vi "探头窗口-24-4列.vi"() -> ()   [LabVIEW 2017]
panel:
  in  "更新数据":T1
  in  "停止信号":bool=TRUE
  out "更新数据？":bool=TRUE
  out "引用-切回列表模式？":refnum<vi>
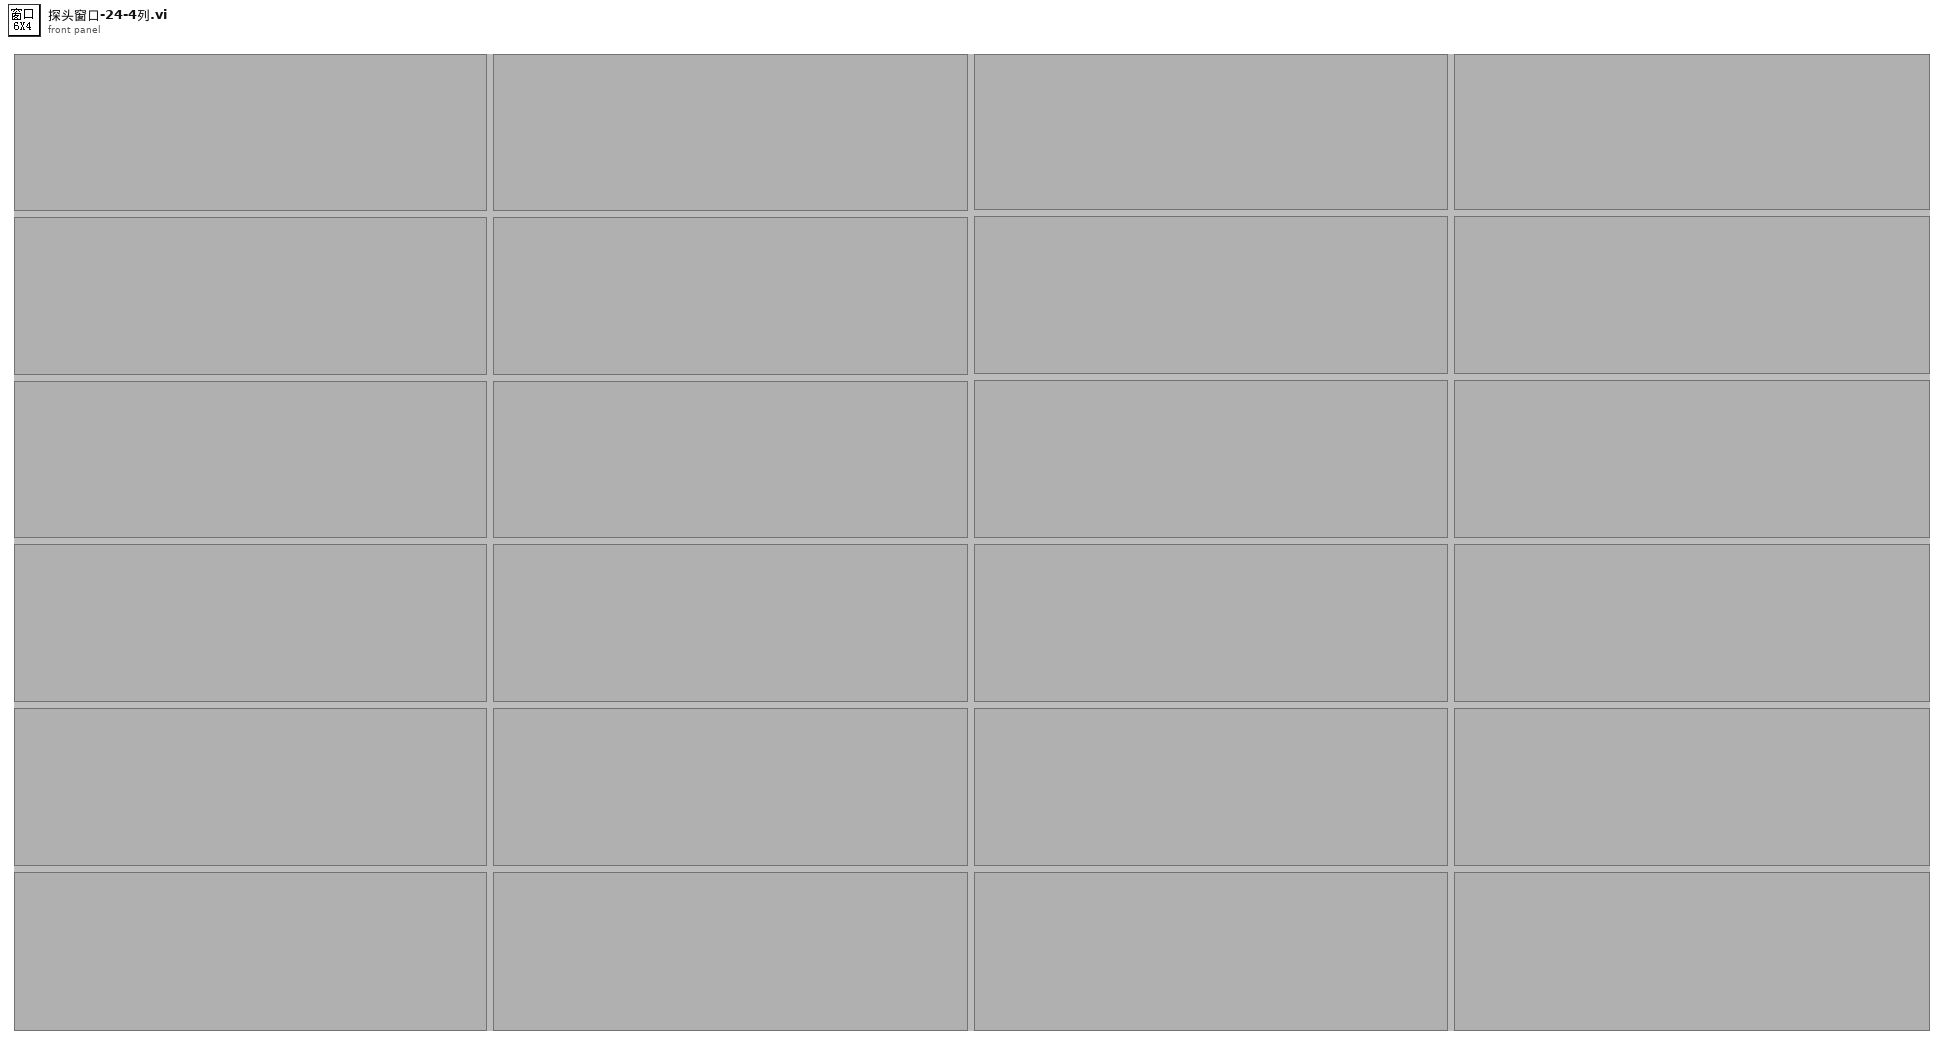
[diagram p1: front panel]
types:
  T1 = cluster{"探头启用状态？":bool[], "测量值":cluster{"X":timestamp, "Y":dbl}[], "限值":cluster{"限值1":dbl, "限值2":dbl, "探头限值":enum16{"一级限值", "二级限值"}}[], "报警状态":enum16{"正常", "一级报警", "二级报警", "累积报警"}[], "探头信息":string[], "累积剂量":cluster{"设备名称":string, "启用累积？":bool, "起始时间":timestamp, "累积剂量":dbl, "累积报警阈值":dbl}[]}
  T2 = cluster{"启用状态？":bool, "测量值":cluster{"X":timestamp, "Y":dbl}, "限值簇":cluster{"限值1":dbl, "限值2":dbl, "探头限值":enum16{"一级限值", "二级限值"}}, "报警状态":enum16{"正常", "一级报警", "二级报警", "累积报警"}, "探头信息":string, "探头地址":i32, "累积剂量":cluster{"设备名称":string, "启用累积？":bool, "起始时间":timestamp, "累积剂量":dbl, "累积报警阈值":dbl}}
  T3 = typedef "eventvkey.ctl" = enum16{"ASCII", "Enter", "Return", "Shift", "Ctrl", "Alt", "Cmd", "Opt", "Caps", "NumLock", "Clear", "Break", "Up", "Down", "Left", "Right", "Insert", "Delete", "Home", "End", "PageUp", "PageDown", "Escape", "Help", "Pause", "ScrollLock", "F1", "F2", "F3", "F4", "F5", "F6", "F7", "F8", "F9", "F10", "F11", "F12", "F13", "F14", "F15", "F16", "F17", "F18", "F19", "F20", "F21", "F22", "F23", "F24", "Play", "VolumeUp", "VolumeDown", "Mute", "Two Byte Char"}
  T4 = cluster{"限值1":dbl, "限值2":dbl, "探头限值":enum16{"一级限值", "二级限值"}}
  T5 = cluster{"限值1":dbl, "限值2":dbl, "探头限值":enum16{"一级限值", "二级限值"}}[]
  T6 = cluster{"设备名称":string, "启用累积？":bool, "起始时间":timestamp, "累积剂量":dbl, "累积报警阈值":dbl}[]
  T7 = cluster{"设备名称":string, "启用累积？":bool, "起始时间":timestamp, "累积剂量":dbl, "累积报警阈值":dbl}
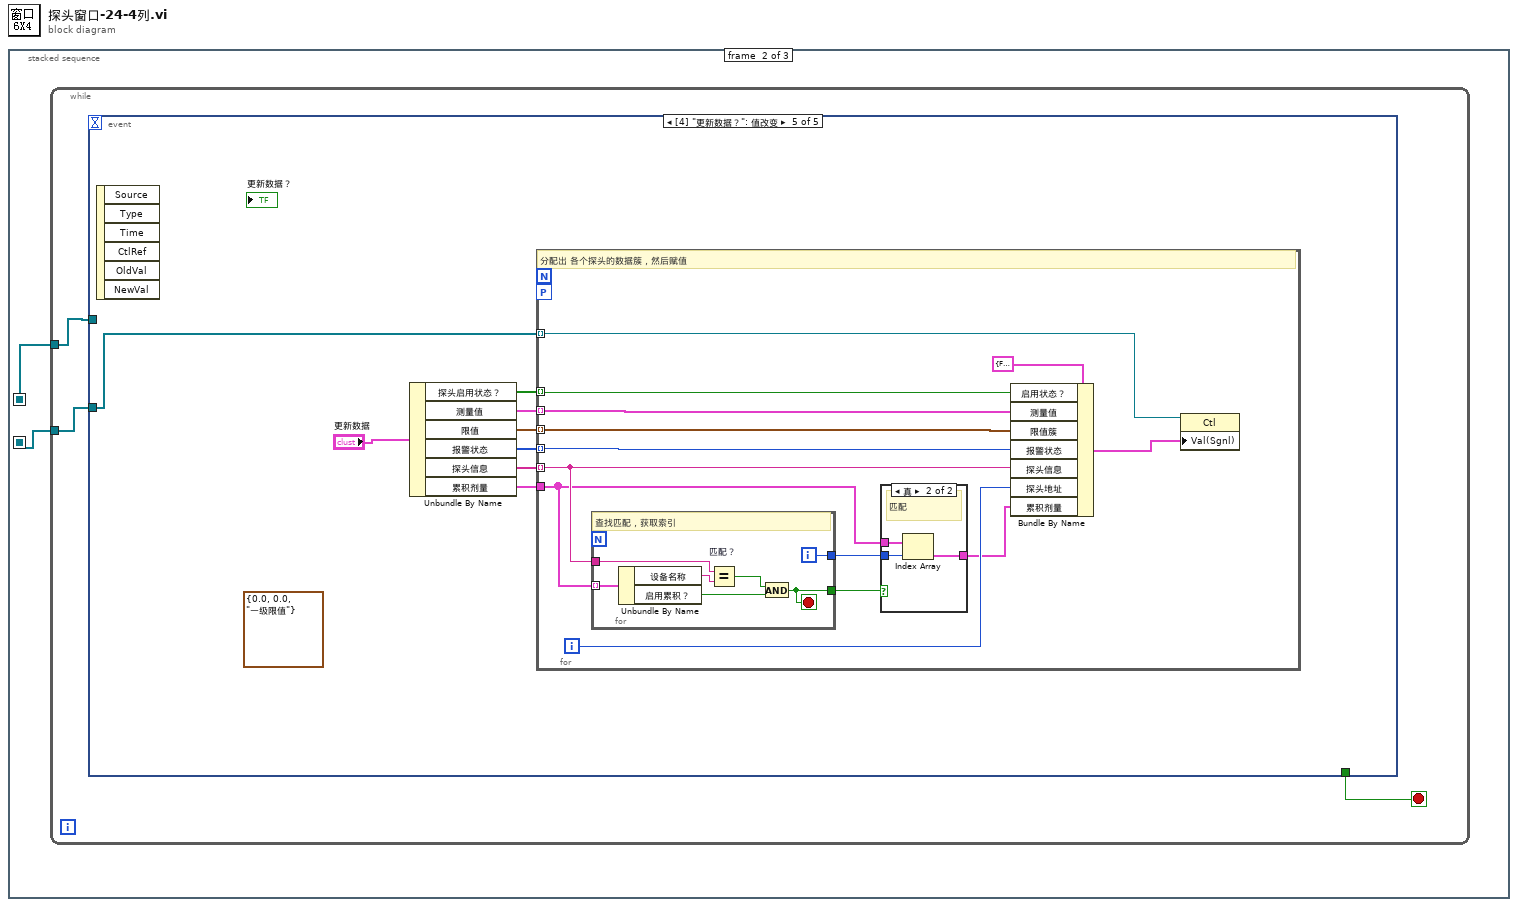
[diagram p0: block diagram]
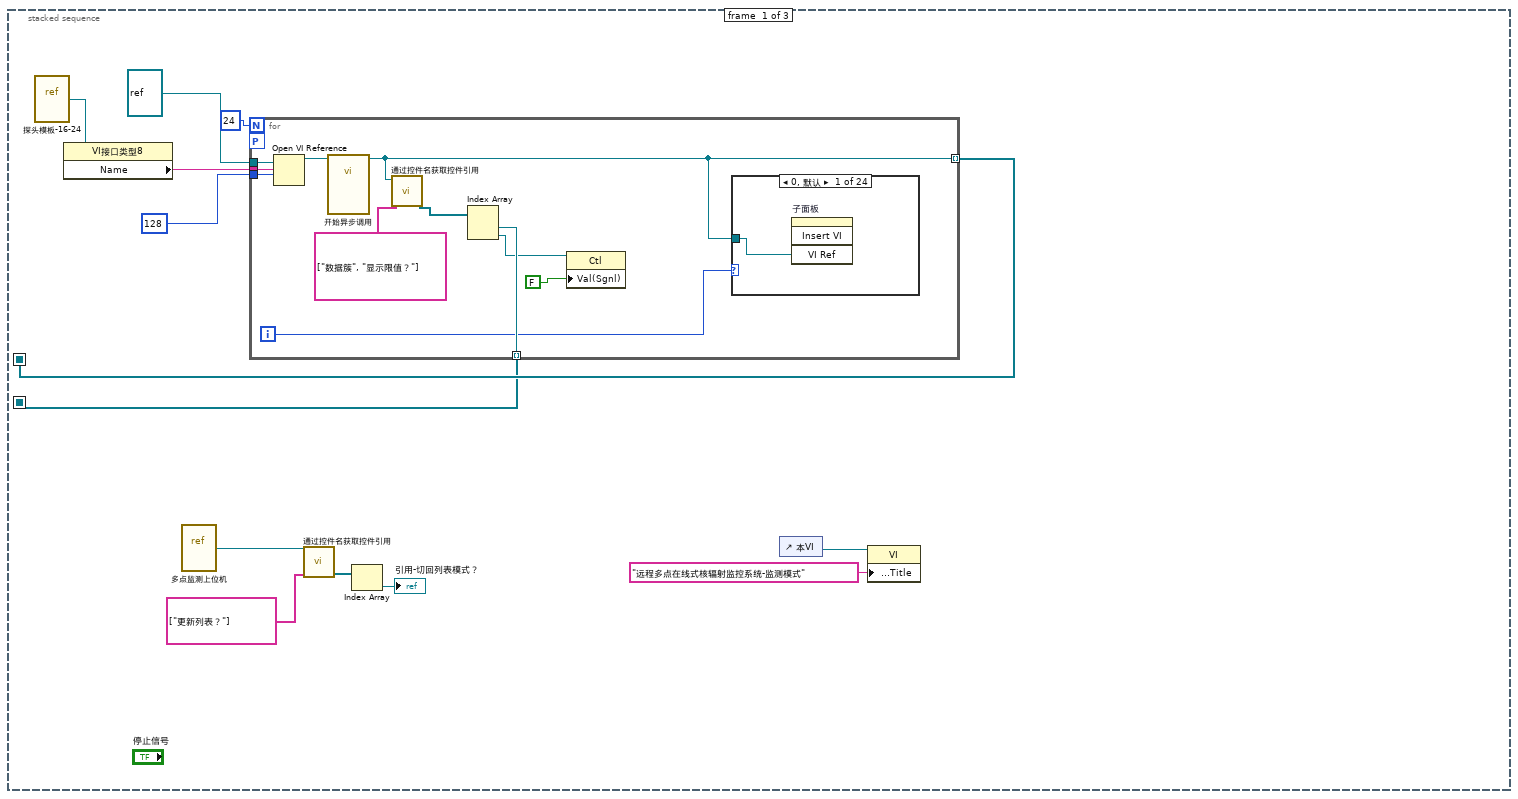
[diagram p2: hidden frame]
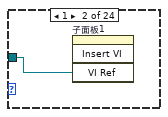
[diagram p3: hidden frame]
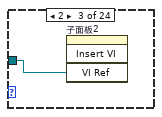
[diagram p4: hidden frame]
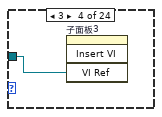
[diagram p5: hidden frame]
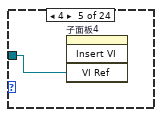
[diagram p6: hidden frame]
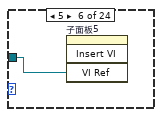
[diagram p7: hidden frame]
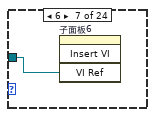
[diagram p8: hidden frame]
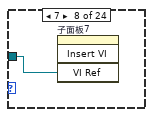
[diagram p9: hidden frame]
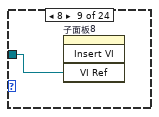
[diagram p10: hidden frame]
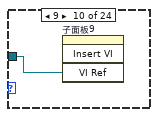
[diagram p11: hidden frame]
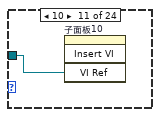
[diagram p12: hidden frame]
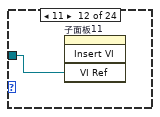
[diagram p13: hidden frame]
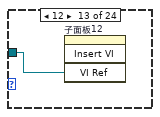
[diagram p14: hidden frame]
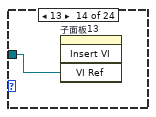
[diagram p15: hidden frame]
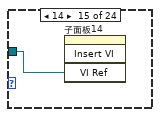
[diagram p16: hidden frame]
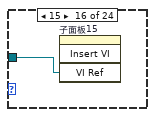
[diagram p17: hidden frame]
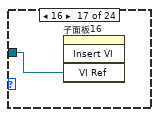
[diagram p18: hidden frame]
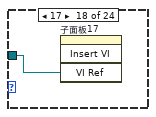
[diagram p19: hidden frame]
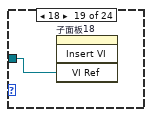
[diagram p20: hidden frame]
diagram:
  n1 = stacked-sequence {
    seq-local: [w8 _ _] -> [_ w50 _]
    seq-local: [w7 _ _] -> [_ w49 _]
    frame #0 {
      n2 = vi-ref "探头模板-16-24.vi"() -> (w13:refnum<vi>)
      n3 = property class="VI接口类型8"(reference=w13) -> ("Name"=w12:string)  [unwired: 1 in, 2 out]
      n4 = vi-ref "多点监测上位机.vi"() -> (w3:refnum<vi>)
      n5 = for {
        N: 24 -> [_]
        tunnel: w12 -> [w24]
        tunnel: 128 ("选项") -> [w23]
        tunnel: refnum<vi> refnum ("类型说明符VI引用句柄（仅用于类型）") -> [w22]
        tunnel: [w16] -> w8 mode=indexing
        tunnel: [w19] -> w7 mode=indexing
        workers-P: _ -> [_]
        i -> [w18]
        n6 = Open VI Reference(type specifier VI Refnum (for type only)=w22, vi path=w24, options=w23) -> (vi reference=w17:refnum<vi>)  [unwired: 3 in, 1 out]
        n7 = call-by-ref "开始异步调用"(reference=w17) -> (reference out=w16:refnum<vi>)  [unwired: 13 in, 1 out]
        n8 = call "通过控件名获取控件引用.vi"("控件名数组"=string[] ["数据簇", "显示限值？"], "VI引用"=w16) -> ("控件引用输出"=w21:refnum<vi>[])  [unwired: 7 in, 2 out]
        n9 = Index Array(array=w21) -> (element #1=w19:refnum<vi>, element #2=w15:refnum<vi>)  [unwired: 2 in]
        n10 = property class="Ctl"(reference=w15, "Val(Sgnl)"=FALSE ("显示报警限值？")) -> ()  [unwired: 1 in, 2 out]
        n11 = case shown="0, 默认" w18 {
          tunnel: w16 -> [w25 w26 w27 w28 w29 w30 w31 w32 w33 w34 w35 w36 w37 w38 w39 w40 w41 w42 w43 w44 w45 w46 w47 w48]
          frame 0, Default {
            n12 = invoke on="子面板" class="子面板" method="Insert VI"("VI Ref"=w25) -> ()  [unwired: 3 in, 4 out]
          }
          frame 1 {
            n13 = invoke on="子面板1" class="SubPnl" method="Insert VI"("VI Ref"=w26) -> ()  [unwired: 3 in, 4 out]
          }
          frame 2 {
            n14 = invoke on="子面板2" class="SubPnl" method="Insert VI"("VI Ref"=w27) -> ()  [unwired: 3 in, 4 out]
          }
          frame 3 {
            n15 = invoke on="子面板3" class="SubPnl" method="Insert VI"("VI Ref"=w28) -> ()  [unwired: 3 in, 4 out]
          }
          frame 4 {
            n16 = invoke on="子面板4" class="SubPnl" method="Insert VI"("VI Ref"=w29) -> ()  [unwired: 3 in, 4 out]
          }
          frame 5 {
            n17 = invoke on="子面板5" class="SubPnl" method="Insert VI"("VI Ref"=w30) -> ()  [unwired: 3 in, 4 out]
          }
          frame 6 {
            n18 = invoke on="子面板6" class="SubPnl" method="Insert VI"("VI Ref"=w31) -> ()  [unwired: 3 in, 4 out]
          }
          frame 7 {
            n19 = invoke on="子面板7" class="SubPnl" method="Insert VI"("VI Ref"=w32) -> ()  [unwired: 3 in, 4 out]
          }
          frame 8 {
            n20 = invoke on="子面板8" class="SubPnl" method="Insert VI"("VI Ref"=w33) -> ()  [unwired: 3 in, 4 out]
          }
          frame 9 {
            n21 = invoke on="子面板9" class="SubPnl" method="Insert VI"("VI Ref"=w34) -> ()  [unwired: 3 in, 4 out]
          }
          frame 10 {
            n22 = invoke on="子面板10" class="SubPnl" method="Insert VI"("VI Ref"=w35) -> ()  [unwired: 3 in, 4 out]
          }
          frame 11 {
            n23 = invoke on="子面板11" class="SubPnl" method="Insert VI"("VI Ref"=w36) -> ()  [unwired: 3 in, 4 out]
          }
          frame 12 {
            n24 = invoke on="子面板12" class="SubPnl" method="Insert VI"("VI Ref"=w37) -> ()  [unwired: 3 in, 4 out]
          }
          frame 13 {
            n25 = invoke on="子面板13" class="SubPnl" method="Insert VI"("VI Ref"=w38) -> ()  [unwired: 3 in, 4 out]
          }
          frame 14 {
            n26 = invoke on="子面板14" class="SubPnl" method="Insert VI"("VI Ref"=w39) -> ()  [unwired: 3 in, 4 out]
          }
          frame 15 {
            n27 = invoke on="子面板15" class="SubPnl" method="Insert VI"("VI Ref"=w40) -> ()  [unwired: 3 in, 4 out]
          }
          frame 16 {
            n28 = invoke on="子面板16" class="SubPnl" method="Insert VI"("VI Ref"=w41) -> ()  [unwired: 3 in, 4 out]
          }
          frame 17 {
            n29 = invoke on="子面板17" class="SubPnl" method="Insert VI"("VI Ref"=w42) -> ()  [unwired: 3 in, 4 out]
          }
          frame 18 {
            n30 = invoke on="子面板18" class="SubPnl" method="Insert VI"("VI Ref"=w43) -> ()  [unwired: 3 in, 4 out]
          }
          frame 19 {
            n31 = invoke on="子面板19" class="SubPnl" method="Insert VI"("VI Ref"=w44) -> ()  [unwired: 3 in, 4 out]
          }
          frame 20 {
            n32 = invoke on="子面板20" class="SubPnl" method="Insert VI"("VI Ref"=w45) -> ()  [unwired: 3 in, 4 out]
          }
          frame 21 {
            n33 = invoke on="子面板21" class="SubPnl" method="Insert VI"("VI Ref"=w46) -> ()  [unwired: 3 in, 4 out]
          }
          frame 22 {
            n34 = invoke on="子面板22" class="SubPnl" method="Insert VI"("VI Ref"=w47) -> ()  [unwired: 3 in, 4 out]
          }
          frame 23 {
            n35 = invoke on="子面板23" class="SubPnl" method="Insert VI"("VI Ref"=w48) -> ()  [unwired: 3 in, 4 out]
          }
        }
      }
      n36 = call "通过控件名获取控件引用.vi"("控件名数组"=string[] ["更新列表？"], "VI引用"=w3) -> ("控件引用输出"=w5:refnum<vi>[])  [unwired: 7 in, 2 out]
      n37 = Index Array(array=w5) -> (element=→"引用-切回列表模式？":refnum<vi>)  [unwired: 1 in]
      n38 = control-ref of="本VI"() -> (w2:refnum<vi>)
      n39 = property class="VI"(reference=w2, "Front Panel.Title"="远程多点在线式核辐射监控系统-监测模式" ("前面板窗口:标题")) -> ()  [unwired: 1 in, 2 out]
    }
    frame #1 {
      n40 = while {
        tunnel: w50 -> [w52]
        tunnel: w49 -> [w51]
        stop <- w53 stop-if-true
        n41 = event shown="[4] \"更新数据？\": 值改变" {
          selector: _ -> [_ _ _ _ _]
          dyn-events: _ -> [_ _ _ _ _]
          timeout: _ -> [_ _ _ _ _]
          tunnel: [_ TRUE ("放弃？") _ _ _] -> w53
          tunnel: w52 -> [_ w57 _ _ _]
          tunnel: w51 -> [_ _ _ _ w65]
          event Timeout {
            n42 = event-data() -> ()  [unwired: 1 in, 3 out]
          }
          event "停止信号": Value Change {
            w56 = TRUE  # T
            n43 = event-data() -> ()  [unwired: 1 in, 6 out]
            n44 = for {
              tunnel: w57 -> [w61] mode=indexing
              workers-P: _ -> [_]
              n45 = invoke class="VI (严格)" method="Abort VI"(reference=w61) -> (reference out=w59:refnum<vi>, error out=w60:errorcluster)  [unwired: 2 in, 1 out]
              n46 = Close Reference(reference=w59, error in (no error)=w60) -> (error out=w58:errorcluster)
              n47 = call <vilib>:"Clear Errors.vi"("error in (no error)"=w58) -> ()  [unwired: 5 in, 2 out]
            }
            n48 = local read "引用-切回列表模式？"() -> (w55:refnum<vi>)
            n49 = property class="Ctl"(reference=w55, "Val(Sgnl)"=w56) -> ()  [unwired: 1 in, 2 out]
          }
          event Panel Close? {
            n50 = event-data() -> ()  [unwired: 1 in, 4 out]
            n51 = property on="停止信号" class="Bool (严格)"("Val(Sgnl)"=TRUE ("值(信号)")) -> ()  [unwired: 2 in, 2 out]
            n52 = event-data() -> ()  [unwired: 2 in, 1 out]
          }
          event Key Down {
            n53 = event-data() -> ("VKey"=w63:T3)  [unwired: 1 in, 9 out]
            n54 = case shown="\"Enter\"" w63 {
              frame "ASCII", Default {
              }
              frame "Enter" {
                w64 = TRUE  # T
                n55 = property on="停止信号" class="Bool (严格)"("Val(Sgnl)"=w64) -> ()  [unwired: 2 in, 2 out]
              }
            }
          }
          event "更新数据？": Value Change {
            (unwired) T4 {"限值1"=0.0, "限值2"=0.0, "探头限值"=enum."一级限值"} ("探头限值簇")
            n56 = event-data() -> ()  [unwired: 1 in, 6 out]
            n57 = Unbundle By Name("更新数据") -> ("探头启用状态？"=w66:bool[], "测量值"=w67:cluster{"X":timestamp, "Y":dbl}[], "限值"=w68:T5, "报警状态"=w69:enum16{"正常", "一级报警", "二级报警", "累积报警"}[], "探头信息"=w70:string[], "累积剂量"=w71:T6)
            n58 = for {
              tunnel: w66 -> [w85] mode=indexing
              tunnel: w67 -> [w84] mode=indexing
              tunnel: w68 -> [w83] mode=indexing
              tunnel: w69 -> [w82] mode=indexing
              tunnel: w70 -> [w77] mode=indexing
              workers-P: _ -> [_]
              tunnel: w65 -> [w80] mode=indexing
              tunnel: w71 -> [w76]
              i -> [w78]
              # "分配出 各个探头的数据簇，然后赋值"
              n59 = for {
                tunnel: w76 -> [w95] mode=indexing
                tunnel: w77 -> [w93]
                tunnel: [w90] -> w75
                tunnel: [w89] -> w74
                i -> [w90]
                stop <- w89 stop-if-true
                # "查找匹配，获取索引"
                n60 = Unbundle By Name(w95) -> ("设备名称"=w94:string, "启用累积？"=w91:bool)
                n61 = Equal? "匹配？"(x=w93, y=w94) -> (x = y?=w92:bool)
                n62 = And(x=w92, y=w91) -> (x .and. y?=w89:bool)
              }
              n63 = case shown="真" w74 {
                tunnel: w76 -> [_ w88]
                tunnel: w75 -> [_ w87]
                tunnel: [_ w86] -> w73
                frame False {
                  # "不匹配"
                }
                frame True {
                  # "匹配"
                  n64 = Index Array(array=w88, index=w87) -> (element=w86:T7)
                }
              }
              n65 = Bundle By Name(cluster=T2 {"启用状态？"=FALSE, "测量值"={"X"=timestamp(0 s since 1904-01-01), "Y"=0.0}, "限值簇"={"限值1"=0.0, "限值2"=0.0, "探头限值"=enum."一级限值"}, "报警状态"=enum."正常", "探头信息"="", "探头地址"=0, "累积剂量"={"设备名称"="", "启用累积？"=FALSE, "起始时间"=timestamp(0 s since 1904-01-01), "累积剂量"=0.0, "累积报警阈值"=0.0}} ("输出簇"), "启用状态？"=w85, "测量值"=w84, "限值簇"=w83, "报警状态"=w82, "探头信息"=w77, "探头地址"=w78, "累积剂量"=w73) -> (w79:T2)
              n66 = property class="Ctl"(reference=w80, "Val(Sgnl)"=w79) -> ()  [unwired: 1 in, 2 out]
            }
          }
        }
      }
    }
    frame #2 {
      n67 = control-ref of="本VI"() -> (w99:refnum<vi>)
      n68 = invoke class="VI" method="FP.Close"(reference=w99) -> (reference out=w98:refnum<vi>, error out=w97:errorcluster)  [unwired: 2 in, 1 out]
      n69 = invoke class="VI" method="Abort VI"(reference=w98, error in=w97) -> (error out=w96:errorcluster)  [unwired: 1 in, 2 out]
      n70 = call <vilib>:"Clear Errors.vi"("error in (no error)"=w96) -> ()  [unwired: 5 in, 2 out]
    }
  }
